vi "SL9200_CMD.vi"(0 "Address":string="01", 1 "Mode":enum16{"Read", "Write"}(ring), 5 "Command":T2=49 items=["Heat_Flow", "Mass_Flow", "Corrected_Volume_Flow", "Volume_Flow", "Temperature", "Temperature2", "Delta_Temperature", "Pressure", "Diff_Pressure", "Density", "Spec_Enthalpy", "Date", "Time", "Level", "Peak_Demand", "Demand_Last_Hour", "Peak_Demand_Time", "Peak_Demand_Date", "Viscosity", "Reynolds_Number", "Heat_Total", "Grand_Heat_Total", "Mass_Total", "Grand_Mass", "Corrected_Volume_Total", "Grand_Corrected_Volume", "Volume_Total", "Grand_Volume", "Totalizer_Reset", "Alarm_Reset", "Barometric", "Fluid_Type", "Reference_Density", "Therm_Expansion_Coef", "Combustion_Heat", "Specific_Heat", "Flow_Z_Factor", "Ref_Z_Factor", "Isentropic_Exponent", "Viscosity_A", "Viscosity_B", "Reference_Temperature", "Calibration_Density", "Base_Density_H2O_4C", "Per_Mole_N2", "Per_Mole_CO2", "Tag_Number", "Software_Version", "Hardware_Version", "Order_Code", "Serial_Number", "Sensor_Serial_Num"], 7 "Write Data":string="0000") -> (6 "Command String":string)   [LabVIEW 2009]
uses:
  SL9200_Registers.ctl
panel:
  in  "string":string="V"
  in  "Commands":T1(array[cluster])=[{"Command Name"="Heat_Flow", "Registers"="00,00"}, {"Command Name"="Mass_Flow", "Registers"="00,01"}, {"Command Name"="Corrected_Volume_Flow", "Registers"="00,02"}, {"Command Name"="Volume_Flow", "Registers"="00,03"}, {"Command Name"="Temperature", "Registers"="00,04"}, {"Command Name"="Temperature2", "Registers"="00,05"}, {"Command Name"="Delta_Temperature", "Registers"="00,06"}, {"Command Name"="Pressure", "Registers"="00,07"}, {"Command Name"="Diff_Pressure", "Registers"="00,08"}, {"Command Name"="Density", "Registers"="00,09"}, {"Command Name"="Spec_Enthalpy", "Registers"="00,10"}, {"Command Name"="Date", "Registers"="00,11"}, {"Command Name"="Time", "Registers"="00,12"}, {"Command Name"="Level", "Registers"="00,15"}, {"Command Name"="Peak_Demand", "Registers"="00,16"}, {"Command Name"="Demand_Last_Hour", "Registers"="00,17"}, {"Command Name"="Peak_Demand_Time", "Registers"="00,18"}, {"Command Name"="Peak_Demand_Date", "Registers"="00,19"}, {"Command Name"="Viscosity", "Registers"="00,20"}, {"Command Name"="Reynolds_Number", "Registers"="00,21"}, {"Command Name"="Heat_Total", "Registers"="01,00"}, {"Command Name"="Grand_Heat_Total", "Registers"="01,01"}, {"Command Name"="Mass_Total", "Registers"="01,02"}, {"Command Name"="Grand_Mass", "Registers"="01,03"}, {"Command Name"="Corrected_Volume_Total", "Registers"="01,04"}, {"Command Name"="Grand_Corrected_Volume", "Registers"="01,05"}, {"Command Name"="Volume_Total", "Registers"="01,06"}, {"Command Name"="Grand_Volume", "Registers"="01,07"}, {"Command Name"="Totalizer_Reset", "Registers"="03,08"}, {"Command Name"="Alarm_Reset", "Registers"="03,09"}, {"Command Name"="Barometric", "Registers"="08,08"}, {"Command Name"="Fluid_Type", "Registers"="10,01"}, {"Command Name"="Reference_Density", "Registers"="10,02"}, {"Command Name"="Therm_Expansion_Coef", "Registers"="10,03"}, {"Command Name"="Combustion_Heat", "Registers"="10,04"}, {"Command Name"="Specific_Heat", "Registers"="10,05"}, {"Command Name"="Flow_Z_Factor", "Registers"="10,06"}, {"Command Name"="Ref_Z_Factor", "Registers"="10,07"}, {"Command Name"="Isentropic_Exponent", "Registers"="10,08"}, {"Command Name"="Viscosity_A", "Registers"="10,09"}, {"Command Name"="Viscosity_B", "Registers"="10,10"}, {"Command Name"="Reference_Temperature", "Registers"="10,11"}, {"Command Name"="Calibration_Density", "Registers"="10,12"}, {"Command Name"="Base_Density_H2O_4C", "Registers"="10,13"}, {"Command Name"="Per_Mole_N2", "Registers"="10,14"}, {"Command Name"="Per_Mole_CO2", "Registers"="10,15"}, {"Command Name"="Tag_Number", "Registers"="19,00"}, {"Command Name"="Software_Version", "Registers"="19,01"}, {"Command Name"="Hardware_Version", "Registers"="19,02"}, {"Command Name"="Order_Code", "Registers"="19,03"}, {"Command Name"="Serial_Number", "Registers"="19,04"}, {"Command Name"="Sensor_Serial_Num", "Registers"="19,05"}]
  out "Data Array":string[][](array[string])=[["Heat_Flow", "00,00", "R", "R/W", "R", "n/a", "n/a", "SL92", ""], ["Mass_Flow", "00,01", "R", "R/W", "R", "n/a", "n/a", "SL91/All", ""], ["Corrected_Volume_Flow", "00,02", "R", "R/W", "R", "n/a", "n/a", "SL91/All", ""], ["Volume_Flow", "00,03", "R", "R/W", "R", "n/a", "n/a", "SL91/All", ""], ["Temperature", "00,04", "R", "R/W", "R", "n/a", "n/a", "SL91/All", ""], ["Temperature2", "00,05", "R", "R/W", "R", "n/a", "n/a", "All", ""], ["Delta_Temperature", "00,06", "R", "R/W", "R", "n/a", "n/a", "All", ""], ["Pressure", "00,07", "R", "R/W", "R", "n/a", "n/a", "All", ""], ["Diff_Pressure", "00,08", "R", "R/W", "R", "n/a", "n/a", "All", ""], ["Density", "00,09", "R", "R/W", "R", "n/a", "n/a", "SL91/All", ""], ["Spec_Enthalpy", "00,10", "R", "R/W", "R", "n/a", "n/a", "All", ""], ["Date", "00,11", "R", "R", "R", "n/a", "n/a", "SL91/All", ""], ["Time", "00,12", "R", "R", "R", "n/a", "n/a", "SL91/All", ""], ["Level", "00,15", "R", "R", "R", "n/a", "n/a", "N/A", ""], ["Peak_Demand", "00,16", "R", "R", "R", "n/a", "n/a", "SL92", ""], ["Demand_Last_Hour", "00,17", "R", "R", "R", "n/a", "n/a", "SL92", ""], ["Peak_Demand_Time", "00,18", "R", "R", "R", "n/a", "n/a", "SL92", ""], ["Peak_Demand_Date", "00,19", "R", "R", "R", "n/a", "n/a", "SL92", ""], ["Viscosity", "00,20", "R", "R", "R", "n/a", "n/a", "N/A", ""], ["Reynolds_Number", "00,21", "R", "R", "R", "n/a", "n/a", "N/A", ""], ["Heat_Total", "01,00", "R", "R/W", "R", "n/a", "n/a", "All", ""], ["Grand_Heat_Total", "01,01", "R", "R/W", "R", "n/a", "n/a", "All", ""], ["Mass_Total", "01,02", "R", "R/W", "R", "n/a", "n/a", "SL91/All", ""], ["Grand_Mass", "01,03", "R", "R/W", "R", "n/a", "n/a", "SL91/All", ""], ["Corrected_Volume_Total", "01,04", "R", "R/W", "R", "n/a", "n/a", "SL91/All", ""], ["Grand_Corrected_Volume", "01,05", "R", "R/W", "R", "n/a", "n/a", "SL91/All", ""], ["Volume_Total", "01,06", "R", "R/W", "R", "n/a", "n/a", "SL91/All", ""], ["Grand_Volume", "01,07", "R", "R/W", "R", "n/a", "n/a", "SL91/All", ""], ["Totalizer_Reset", "03,08", "", "", "", "", "", "", ""], ["Alarm_Reset", "03,09", "", "", "", "", "", "", ""], ["Barometric", "08,08", "", "", "", "", "", "", ""], ["Fluid_Type", "10,01", "", "", "", "", "", "", ""], ["Reference_Density", "10,02", "R/W", "R", "R", "n/a", "n/a", "SL91/All", ""], ["Therm_Expansion_Coef", "10,03", "R/W", "R", "R", "n/a", "n/a", "SL91/All", ""], ["Combustion_Heat", "10,04", "R/W", "R", "R", "n/a", "n/a", "SL92", ""], ["Specific_Heat", "10,05", "R/W", "R", "R", "n/a", "n/a", "SL92", ""], ["Flow_Z_Factor", "10,06", "R/W", "R", "R", "n/a", "n/a", "SL92", ""], ["Ref_Z_Factor", "10,07", "R/W", "R", "R", "n/a", "n/a", "SL92", ""], ["Isentropic_Exponent", "10,08", "R/W", "R", "R", "n/a", "n/a", "SL92", ""], ["Viscosity_A", "10,09", "R/W", "R", "R", "n/a", "n/a", "SL91/SL92", ""], ["Viscosity_B", "10,10", "R/W", "R", "R", "n/a", "n/a", "SL91/SL92", ""], ["Reference_Temperature", "10,11", "R/W", "R", "R", "n/a", "n/a", "SL91", ""], ["Calibration_Density", "10,12", "R/W", "R", "R", "n/a", "n/a", "SL91", ""], ["Base_Density_H2O_4C", "10,13", "R/W", "R", "R", "n/a", "n/a", "SL91", ""], ["Per_Mole_N2", "10,14", "R/W", "R", "R", "n/a", "n/a", "SL92", ""], ["Per_Mole_CO2", "10,15", "", "", "", "", "", "", ""], ["Tag_Number", "19,00", "R/W", "R", "n/a", "n/a", "n/a", "SL92", ""], ["Software_Version", "19,01", "R", "R", "n/a", "n/a", "n/a", "SL91", ""], ["Hardware_Version", "19,02", "R/W", "R", "n/a", "n/a", "n/a", "SL92", ""], ["Order_Code", "19,03", "R/W", "R", "n/a", "n/a", "n/a", "SL91/SL92", ""], ["Serial_Number", "19,04", "R/W", "R", "n/a", "n/a", "n/a", "SL91/SL92", ""], ["Sensor_Serial_Num", "19,05", "", "", "", "", "", "", ""]]
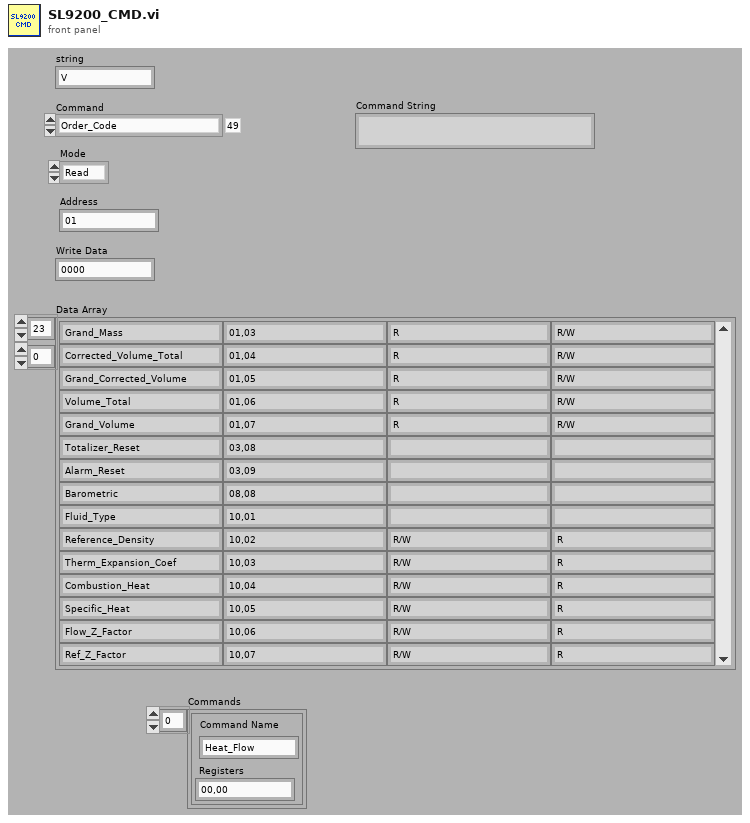
[diagram p1: front panel]
types:
  T1 = cluster{"Command Name":string, "Registers":string}[]
  T2 = typedef "SL9200_Registers.ctl" = u8
  T3 = cluster{"Command Name":string, "Registers":string}
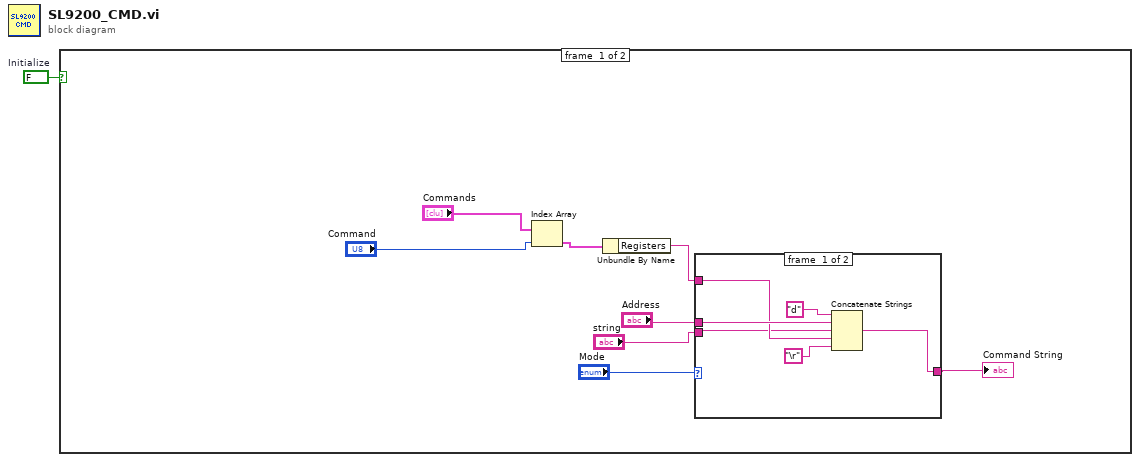
[diagram p0: block diagram]
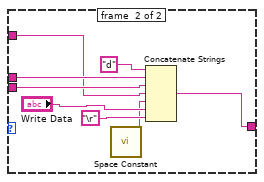
[diagram p2: hidden frame]
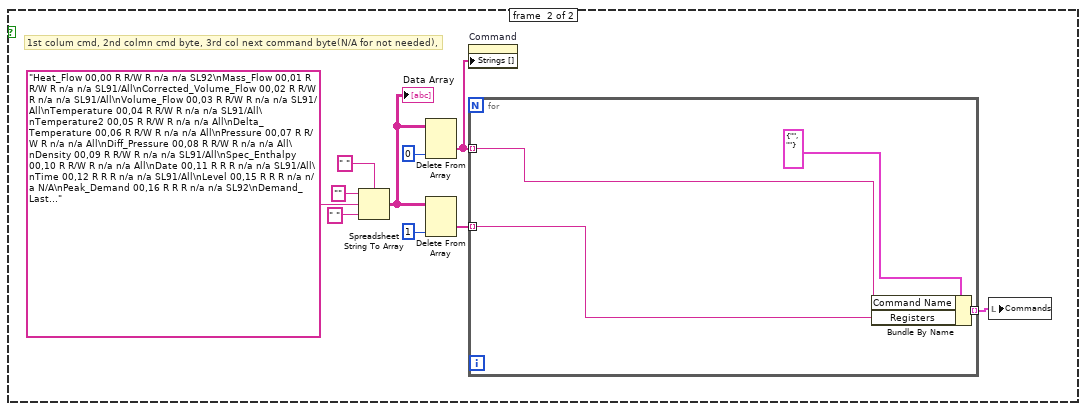
[diagram p3: hidden frame]
diagram:
  w1 = FALSE  # Initialize
  n1 = case shown="False" w1 {
    frame #0 {
      n2 = Index Array(array="Commands", index="Command") -> (element=w7:T3)
      n3 = Unbundle By Name(w7) -> ("Registers"=w2:string)
      n4 = case shown="\"Write\"" "Mode" {
        tunnel: w2 -> [w11 w17]
        tunnel: [w13 w22] -> w3
        tunnel: "Address" -> [w12 w21]
        tunnel: "string" -> [w10 w18]
        frame #0 {
          n5 = Concatenate Strings("d" ("string"), w12, w10, w11, "\r") -> (w13:string)
        }
        frame #1 {
          n6 = call <vilib>:"Space Constant.vi"() -> ("String"=w16:string)
          n7 = Concatenate Strings("d" ("string"), w21, w18, w17, w16, "Write Data", "\r") -> (w22:string)
        }
      }
      "Command String" <- w3
    }
    frame #1 {
      # "1st colum cmd, 2nd colmn cmd byte, 3rd col next command byte(N/A for not needed),"
      n8 = Spreadsheet String To Array(delimiter (Tab)=" ", format string="", spreadsheet string="Heat_Flow 00,00 R R/W R n/a n/a SL92\nMass_Flow 00,01 R R/W R n/a n/a SL91/All\nCorrected_Volume_Flow 00,02 R R/W R n/a n/a SL91/All\nVolume_Flow 00,03 R R/W R n/a n/a SL91/All\nTemperature 00,04 R R/W R n/a n/a SL91/All\nTemperature2 00,05 R R/W R n/a n/a All\nDelta_Temperature 00,06 R R/W R n/a n/a All\nPressure 00,07 R R/W R n/a n/a All\nDiff_Pressure 00,08 R R/W R n/a n/a All\nDensity 00,09 R R/W R n/a n/a SL91/All\nSpec_Enthalpy 00,10 R R/W R n/a n/a All\nDate 00,11 R R R n/a n/a SL91/All\nTime 00,12 R R R n/a n/a SL91/All\nLevel 00,15 R R R n/a n/a N/A\nPeak_Demand 00,16 R R R n/a n/a SL92\nDemand_Last_Hour 00,17 R R R n/a n/a SL92\nPeak_Demand_Time 00,18 R R R n/a n/a SL92\nPeak_Demand_Date 00,19 R R R n/a n/a SL92\nViscosity 00,20 R R R n/a n/a N/A\nReynolds_Number 00,21 R R R n/a n/a N/A\nHeat_Total 01,00 R R/W R n/a n/a All\nGrand_Heat_Total 01,01 R R/W R n/a n/a All\nMass_Total 01,02 R R/W R n/a n/a SL91/All\nGrand_Mass 01,03 R R/W R n/a n/a SL91/All\nCorrected_Volume_Total 01,04 R R/W R n/a n/a SL91/All\nGrand_Corrected_Volume 01,05 R R/W R n/a n/a SL91/All\nVolume_Total 01,06 R R/W R n/a n/a SL91/All\nGrand_Volume 01,07 R R/W R n/a n/a SL91/All\nTotalizer_Reset 03,08\nAlarm_Reset 03,09\nBarometric 08,08\nFluid_Type 10,01\nReference_Density 10,02 R/W R R n/a n/a SL91/All\nTherm_Expansion_Coef 10,03 R/W R R n/a n/a SL91/All\nCombustion_Heat 10,04 R/W R R n/a n/a SL92\nSpecific_Heat 10,05 R/W R R n/a n/a SL92\nFlow_Z_Factor 10,06 R/W R R n/a n/a SL92\nRef_Z_Factor 10,07 R/W R R n/a n/a SL92\nIsentropic_Exponent 10,08 R/W R R n/a n/a SL92\nViscosity_A 10,09 R/W R R n/a n/a SL91/SL92\nViscosity_B 10,10 R/W R R n/a n/a SL91/SL92\nReference_Temperature 10,11 R/W R R n/a n/a SL91\nCalibration_Density 10,12 R/W R R n/a n/a SL91\nBase_Density_H2O_4C 10,13 R/W R R n/a n/a SL91\nPer_Mole_N2 10,14 R/W R R n/a n/a SL92 \nPer_Mole_CO2 10,15\nTag_Number 19,00 R/W R n/a n/a n/a SL92\nSoftware_Version 19,01 R R n/a n/a n/a SL91\nHardware_Version 19,02 R/W R n/a n/a n/a SL92\nOrder_Code 19,03 R/W R n/a n/a n/a SL91/SL92\nSerial_Number 19,04 R/W R n/a n/a n/a SL91/SL92\nSensor_Serial_Num 19,05", array type (2D Dbl)=" " ("delimiter (Tab)")) -> (array=w26:string[][])
      "Data Array" <- w26
      n9 = Delete From Array(array=w26, index (col)=0 ("disabled index (col)")) -> (deleted portion=w29:string[])  [unwired: 2 in, 1 out]
      n10 = Delete From Array(array=w26, index (col)=1 ("disabled index (col)")) -> (deleted portion=w27:string[])  [unwired: 2 in, 1 out]
      n11 = property on="Command" class="Ring (strict)"("Strings []"=w29) -> ()  [unwired: 2 in, 2 out]
      n12 = for {
        tunnel: w29 -> [w37] mode=indexing
        tunnel: w27 -> [w34] mode=indexing
        tunnel: [w36] -> w25 mode=indexing
        n13 = Bundle By Name(cluster=T3 {"Command Name"="", "Registers"=""} ("Cluster"), "Command Name"=w37, "Registers"=w34) -> (w36:T3)
      }
      n14 = local write "Commands"(w25) -> ()
    }
  }
